vi "SIMPS_Get_Mode.vi"(8 "error in (no error)":errorcluster) -> (0 "error out":errorcluster, 3 "String":string)   [LabVIEW 2020]
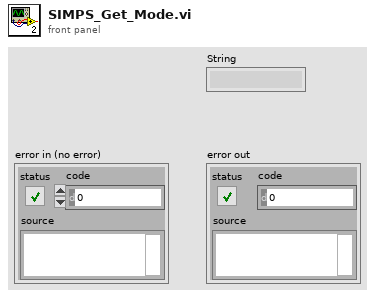
[diagram p1: front panel]
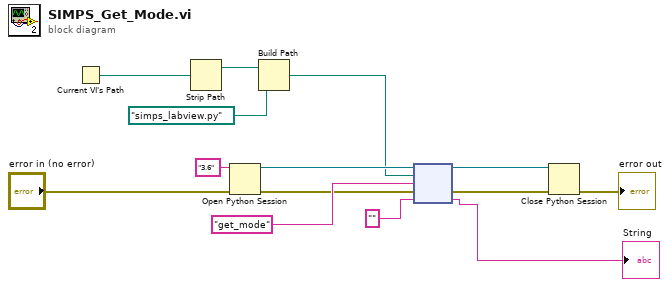
[diagram p0: block diagram]
diagram:
  n1 = Current VI's Path() -> (path=w11:path)
  n2 = Strip Path(path=w11) -> (stripped path=w12:path)  [unwired: 1 out]
  n3 = Open Python Session(python version="3.6" ("Python version"), 3:"error in (no error)") -> (session out=w9:refnum<k35>, error out=w7:errorcluster)  [unwired: 1 in]
  n4 = Build Path(base path=w12, name or relative path=path "simps_labview.py") -> (appended path=w5:path)
  n5 = node(w9, w5, "get_mode" ("function name"), w7, "") -> (w3:refnum<k35>, w2:errorcluster, →"String":string)  [unwired: 2 out]
  n6 = Close Python Session(session in=w3, error in=w2) -> (11:→"error out":errorcluster)
